vi "FRCts20_WebMethods_Redirect_Competition.vi"(7 "response code (200)":i32(ring)=200 items=["100"=100, "101"=101, "200"=200, "201"=201, "202"=202, "203"=203, "204"=204, "205"=205, "206"=206, "300"=300, "301"=301, "302"=302, "303"=303, "304"=304, "305"=305, "306"=306, "307"=307, "400"=400, "401"=401, "402"=402, "403"=403, "404"=404, "405"=405, "406"=406, "407"=407, "408"=408, "409"=409, "410"=410, "411"=411, "412"=412, "413"=413, "414"=414, "415"=415, "416"=416, "417"=417, "500"=500, "501"=501, "502"=502, "503"=503, "504"=504, "505"=505], 8 "error in (no error)":errorcluster, 10 "Single Event":T1, 11 "httpRequestID":u32) -> (0 "error out":errorcluster, 3 "httpRequestID out":u32)   [LabVIEW 2013, in "FRCts20_WebMethods.lvlib"]
uses:
  Web Method Public Interface/FRCts20_WebMethods_ctl_singleEvent.ctl
  Web Method Public Interface/FRCts20_WebMethods_ctl_teamIdentifier.ctl
  FRCts20_WebMethods.lvlib
  <vilib>/wsapi/NI_WebServices.lvlib
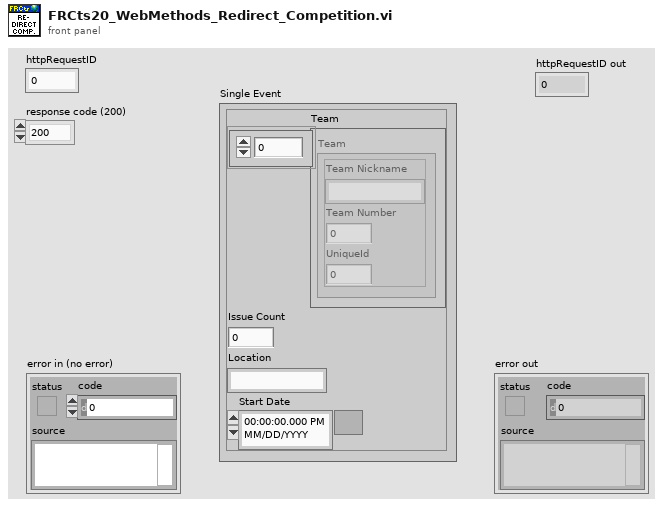
[diagram p1: front panel]
types:
  T1 = typedef "FRCts20_WebMethods.lvlib/FRCts20_WebMethods_ctl_singleEvent.ctl" = cluster{"Team":T2[], "Issue Count":i32, "Location":string, "Start Date ":timestamp}
  T2 = typedef "FRCts20_WebMethods.lvlib/FRCts20_WebMethods_ctl_teamIdentifier.ctl" = cluster{"Team Nickname":string, "Team Number ":u32, "UniqueId":u32}
  T3 = typedef "FRCts20_WebMethods.lvlib/FRCts20_WebMethods_ctl_returntype.ctl" = string
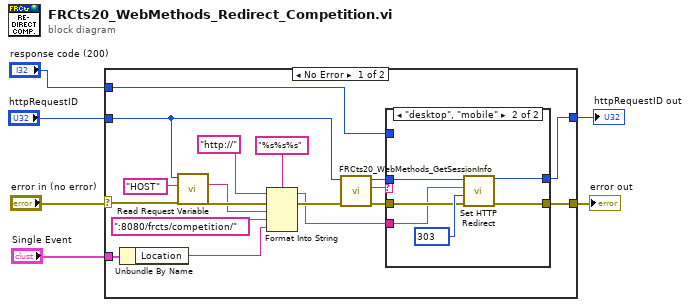
[diagram p0: block diagram]
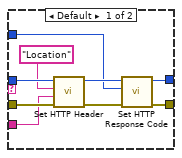
[diagram p2: hidden frame]
diagram:
  n1 = case shown="No Error" "error in (no error)" {
    selector: "error in (no error)" -> [w14 w41]
    tunnel: [w13 w41] -> w6
    tunnel: "httpRequestID" -> [w8 w40]
    tunnel: [w12 w40] -> w4
    tunnel: "Single Event" -> [w24 _]
    tunnel: "response code (200)" -> [w10 _]
    frame No Error {
      n2 = Unbundle By Name(w24) -> ("Location"=w7:string)
      n3 = call <vilib>:"Read Request Variable.vi"("error in (no error)"=w14, "variable name"="HOST", "httpRequestID"=w8) -> ("error out"=w22:errorcluster, "value"=w19:string)  [unwired: 6 in, 1 out]
      n4 = Format Into String(format string="%s%s%s", initial string="http://", error in=w22, w19, ":8080/frcts/competition/", w7) -> (resulting string=w11:string, error out=w15:errorcluster)
      n5 = call "FRCts20_WebMethods_GetSessionInfo.vi"("error in"=w15, "httpRequestID"=w8) -> ("error out"=w17:errorcluster, "Return Type"=w18:T3, "httpRequestID out"=w16:u32)  [unwired: 7 in]
      n6 = case shown="\"desktop\", \"mobile\"" w18 {
        tunnel: [w29 w39] -> w13
        tunnel: [w26 w38] -> w12
        tunnel: w17 -> [w33 w36]
        tunnel: w16 -> [w32 w35]
        tunnel: w11 -> [w30 w34]
        tunnel: w10 -> [w25 _]
        frame Default {
          n7 = call <vilib>:"Set HTTP Header.vi"("error in (no error)"=w33, "header value"=w30, "header"="Location", "httpRequestID"=w32) -> ("error out"=w28:errorcluster, "httpRequestID out"=w27:u32)  [unwired: 6 in]
          n8 = call <vilib>:"Set HTTP Response Code.vi"("error in (no error)"=w28, "response code (200)"=w25, "httpRequestID"=w27) -> ("error out"=w29:errorcluster, "httpRequestID out"=w26:u32)  [unwired: 7 in]
        }
        frame "desktop", "mobile" {
          w37 = 303 items=["100"=100, "101"=101, "200"=200, "201"=201, "202"=202, "203"=203, "204"=204, "205"=205, "206"=206, "300"=300, "301"=301, "302"=302, "303"=303, "304"=304, "305"=305, "306"=306, "307"=307, "400"=400, "401"=401, "402"=402, "403"=403, "404"=404, "405"=405, "406"=406, "407"=407, "408"=408, "409"=409, "410"=410, "411"=411, "412"=412, "413"=413, "414"=414, "415"=415, "416"=416, "417"=417, "500"=500, "501"=501, "502"=502, "503"=503, "504"=504, "505"=505] ("response code (307)")
          n9 = call <vilib>:"Set HTTP Redirect.vi"("error in (no error)"=w36, "response code (307)"=w37, "redirect URL"=w34, "httpRequestID"=w35) -> ("error out"=w39:errorcluster, "httpRequestID out"=w38:u32)  [unwired: 6 in]
        }
      }
    }
    frame Error {
    }
  }
  "error out" <- w6
  "httpRequestID out" <- w4
